vi "_TCP-IP_Q_Bridge._Test_TE.vi"() -> ()   [LabVIEW 2024, in "EQMF.lvlib" / "TCP-IP.lvlib"]
uses:
  TCP-IP.lvlib
  Mgr/TCP-IP Mgr.Config.ctl
  Queues/Queue Utils.lvlib
panel:
  in  "Send Exit to Child":bool=TRUE
  in  "Notification":bool
  out "Con Status":bool
  out "Rcv Cluster":T1={"Enum"=enum."B", "Numeric"=6.0, "Boolean"=TRUE, "String"="ABBCC"}
  in  "Cluster":T1={"Enum"=enum."B", "Numeric"=6.0, "Boolean"=TRUE, "String"="ABBCC"}
  in  "Send Cluster":bool
  in  "Config":T2={"IP"="127.0.0.1", "Port"=8500, "Listener"=FALSE, "Enable"=FALSE}
  out "Connected":bool
  in  "Exit":bool
  out "Rcv Bool":bool
  in  "Send Str":bool
  out "Rcv String":string
  in  "String":string
  in  "Data":bool
  in  "Send Data":bool
  # "Parent"
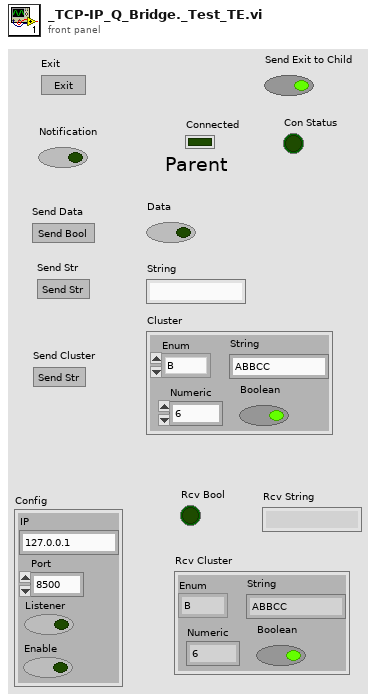
[diagram p1: front panel]
types:
  T1 = cluster{"Enum":enum16{"A", "B", "C"}, "Numeric":dbl, "Boolean":bool, "String":string}
  T2 = typedef "EQMF.lvlib/TCP-IP.lvlib/TCP-IP Mgr.Config.ctl" = cluster{"IP":string, "Port":u16, "Listener":bool, "Enable":bool}
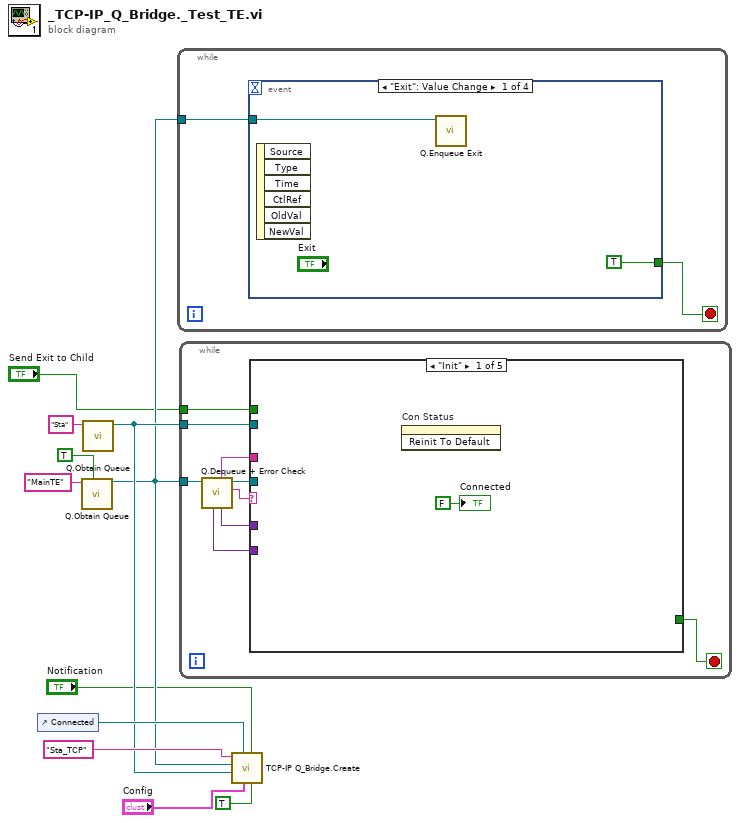
[diagram p0: block diagram]
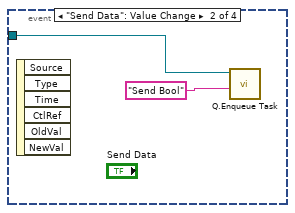
[diagram p2: hidden frame]
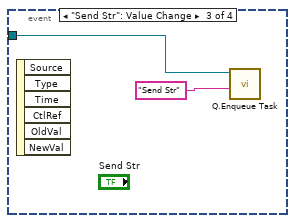
[diagram p3: hidden frame]
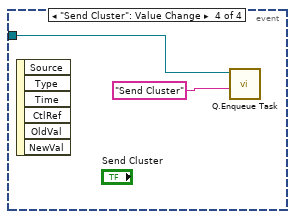
[diagram p4: hidden frame]
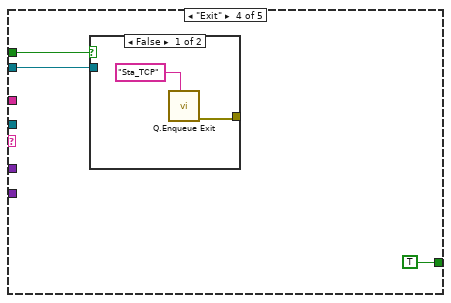
[diagram p7: hidden frame]
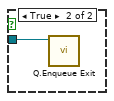
[diagram p8: hidden frame]
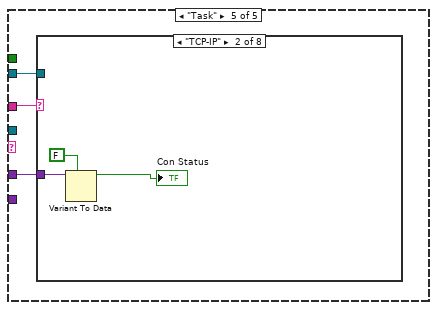
[diagram p9: hidden frame]
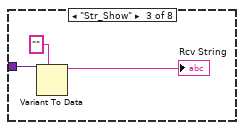
[diagram p11: hidden frame]
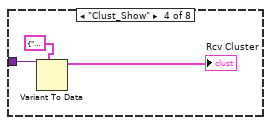
[diagram p12: hidden frame]
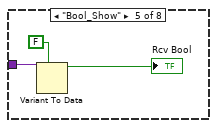
[diagram p13: hidden frame]
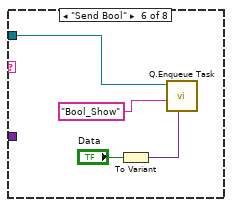
[diagram p14: hidden frame]
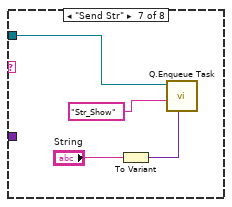
[diagram p15: hidden frame]
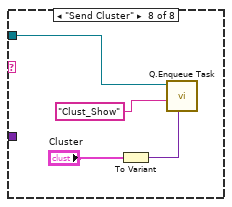
[diagram p16: hidden frame]
diagram:
  n1 = control-ref of="Connected"() -> (w8:refnum<vi>)
  n2 = call "Q.Obtain Queue.vi"("Enqueue Init"=TRUE, "Q Name"="MainTE") -> ("Q Out"=w4:refnum<queue>)  [unwired: 7 in, 2 out]
  n3 = call "Q.Obtain Queue.vi"("Q Name"="Sta") -> ("Q Out"=w5:refnum<queue>)  [unwired: 8 in, 2 out]
  n4 = while {
    tunnel: w4 -> [w13]
    stop <- w12 stop-if-true
    n5 = event shown="[0] \"Exit\": Value Change" {
      selector: _ -> [_ _ _ _]
      dyn-events: _ -> [_ _ _ _]
      timeout: _ -> [_ _ _ _]
      tunnel: w13 -> [w15 w17 w19 w21]
      tunnel: [TRUE _ _ _] -> w12
      event "Exit": Value Change {
        n6 = event-data() -> ()  [unwired: 1 in, 6 out]
        n7 = call "Q.Enqueue Exit.vi"("Q In"=w15) -> ()  [unwired: 9 in, 2 out]
      }
      event "Send Data": Value Change {
        n8 = event-data() -> ()  [unwired: 1 in, 6 out]
        n9 = call "Q.Enqueue Task.vi"("Task Name"="Send Bool", "Q In"=w17) -> ()  [unwired: 8 in, 2 out]
      }
      event "Send Str": Value Change {
        n10 = event-data() -> ()  [unwired: 1 in, 6 out]
        n11 = call "Q.Enqueue Task.vi"("Task Name"="Send Str", "Q In"=w19) -> ()  [unwired: 8 in, 2 out]
      }
      event "Send Cluster": Value Change {
        n12 = event-data() -> ()  [unwired: 1 in, 6 out]
        n13 = call "Q.Enqueue Task.vi"("Task Name"="Send Cluster", "Q In"=w21) -> ()  [unwired: 8 in, 2 out]
      }
    }
  }
  n14 = while {
    tunnel: w4 -> [w29]
    tunnel: w5 -> [w23]
    tunnel: "Send Exit to Child" -> [w22]
    stop <- w24 stop-if-true
    n15 = call "Q.Dequeue + Error Check.vi"("Q In"=w29) -> ("Cmd"=w30:string, "Q Out"=w28:refnum<queue>, "Data1"=w26:variant, "Sub"=w27:string, "Data2"=w25:variant)  [unwired: 5 in, 1 out]
    n16 = case shown="\"Init\"" w30 {
      tunnel: w28 -> [_ _ _ _ _]
      tunnel: w27 -> [_ _ _ _ w40]
      tunnel: w26 -> [_ _ _ _ w39]
      tunnel: w25 -> [_ _ _ _ _]
      tunnel: [_ _ _ TRUE _] -> w24
      tunnel: w23 -> [_ _ _ w33 w38]
      tunnel: w22 -> [_ _ _ w32 _]
      frame "Init" {
        n17 = invoke on="Con Status" class="Bool (strict)" method="Reinit To Default"() -> ()  [unwired: 3 in, 3 out]
        "Connected" <- FALSE ("Connected")
      }
      frame "Reset" {
      }
      frame Default {
      }
      frame "Exit" {
        n18 = case shown="False" w32 {
          tunnel: w33 -> [_ w37]
          tunnel: [w35 _] -> _
          frame False {
            n19 = call "Q.Enqueue Exit.vi"("Q Name"="Sta_TCP") -> ("error out"=w35:errorcluster)  [unwired: 9 in, 1 out]
          }
          frame True {
            n20 = call "Q.Enqueue Exit.vi"("Q In"=w37) -> ()  [unwired: 9 in, 2 out]
          }
        }
      }
      frame "Task" {
        n21 = case shown="\"TCP-IP\"" w40 {
          tunnel: w39 -> [_ w43 w46 w49 w52 _ _ _]
          tunnel: w38 -> [_ _ _ _ _ w56 w60 w64]
          frame Default {
          }
          frame "TCP-IP" {
            n22 = Variant To Data(type=FALSE, Variant=w43) -> (data=→"Con Status":bool)  [unwired: 1 in, 1 out]
          }
          frame "Str_Show" {
            n23 = Variant To Data(type="", Variant=w46) -> (data=→"Rcv String":string)  [unwired: 1 in, 1 out]
          }
          frame "Clust_Show" {
            n24 = Variant To Data(type=T1 {"Enum"=enum."B", "Numeric"=6.0, "Boolean"=TRUE, "String"="ABBCC"} ("Rcv Cluster"), Variant=w49) -> (data=→"Rcv Cluster":T1)  [unwired: 1 in, 1 out]
          }
          frame "Bool_Show" {
            n25 = Variant To Data(type=FALSE, Variant=w52) -> (data=→"Rcv Bool":bool)  [unwired: 1 in, 1 out]
          }
          frame "Send Bool" {
            n26 = To Variant(anything="Data") -> (Variant=w53:variant)
            n27 = call "Q.Enqueue Task.vi"("Data1"=w53, "Task Name"="Bool_Show", "Q In"=w56) -> ()  [unwired: 7 in, 2 out]
          }
          frame "Send Str" {
            n28 = To Variant(anything="String") -> (Variant=w58:variant)
            n29 = call "Q.Enqueue Task.vi"("Data1"=w58, "Task Name"="Str_Show", "Q In"=w60) -> ()  [unwired: 7 in, 2 out]
          }
          frame "Send Cluster" {
            n30 = To Variant(anything="Cluster") -> (Variant=w62:variant)
            n31 = call "Q.Enqueue Task.vi"("Data1"=w62, "Task Name"="Clust_Show", "Q In"=w64) -> ()  [unwired: 7 in, 2 out]
          }
        }
      }
    }
  }
  n32 = call "TCP-IP Q_Bridge.Create.vi"("Auto Exit"=TRUE, "Notification"="Notification", "Config"="Config", "StatusCtrlRef"=w8, "Q_DataOut"=w5, "Q_DataIn"=w4, "Control Q Name"="Sta_TCP" ("Q Name")) -> ()  [unwired: 3 in, 2 out]
